vi "ORS_LinearizeFFTSingleLine - Copy.vi"(2 "Michelson fringes":dbl[](array[numeric]), 4 "Linearization method":u16=1, 5 "inverted Hilbert in":dbl[](array[numeric]), 6 "Use DLL":bool, 7 "RecalFringePhaseFit":dbl[](array[numeric]), 8 "DLL path":path=path "c:/", 12 "Window":T1=62 items=["Rectangle"=0, "Hanning"=1, "Hamming"=2, "Blackman-Harris"=3, "Exact Blackman"=4, "Blackman"=5, "Flat Top"=6, "4 Term B-Harris "=7, "7 Term B-Harris"=8, "Low Sidelobe"=9, "Blackman Nuttall"=11, "Triangle"=30, "Bartlett-Hanning"=31, "Bohman"=32, "Parzen"=33, "Welch"=34, "Kaiser"=60, "Dolph-Chebyshev"=61, "Gaussian"=62], 14 "Linearizer: Interpol. method":i32, 15 "window parameter":dbl=nan, 17 "# zeros added":i32) -> (18 "Output":dbl[](array[numeric]))   [LabVIEW 2016]
uses:
  <vilib>/Analysis/4window.llb/windowTd.ctl
  <vilib>/Analysis/2dsp.llb/Real FFT.vi
  <vilib>/Analysis/4window.llb/Symmetric Window (DBL).vi
  <vilib>/Analysis/2dsp.llb/Zero Padder (DBL).vi
  <vilib>/Analysis/NI_AALPro.lvlib
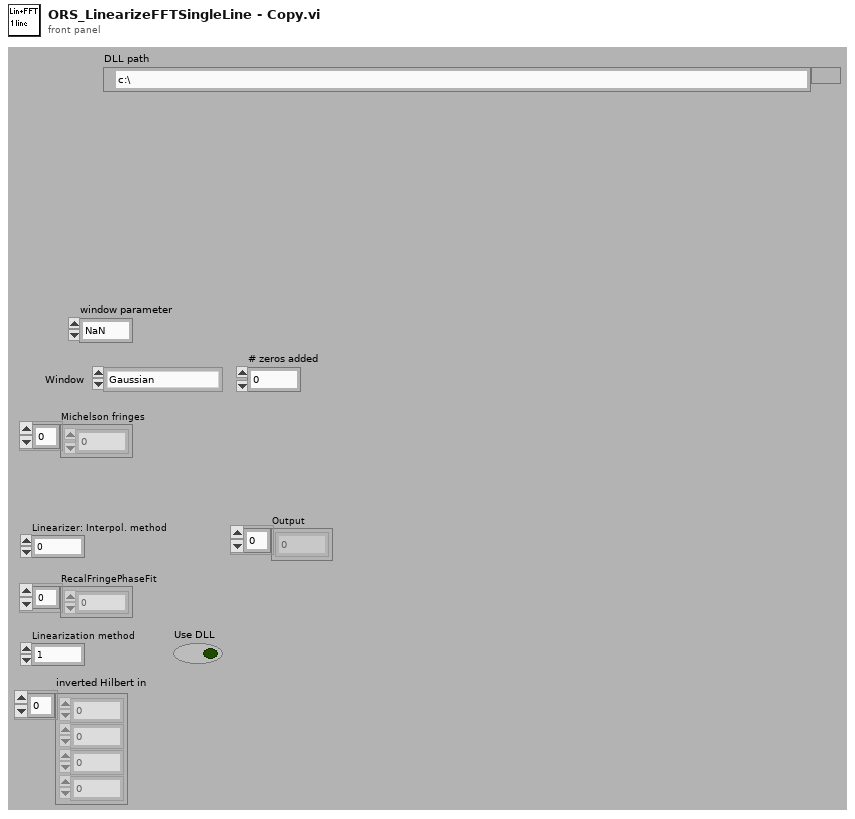
[diagram p1: front panel]
types:
  T1 = typedef "NI_AALPro.lvlib/windowTd.ctl" = u32
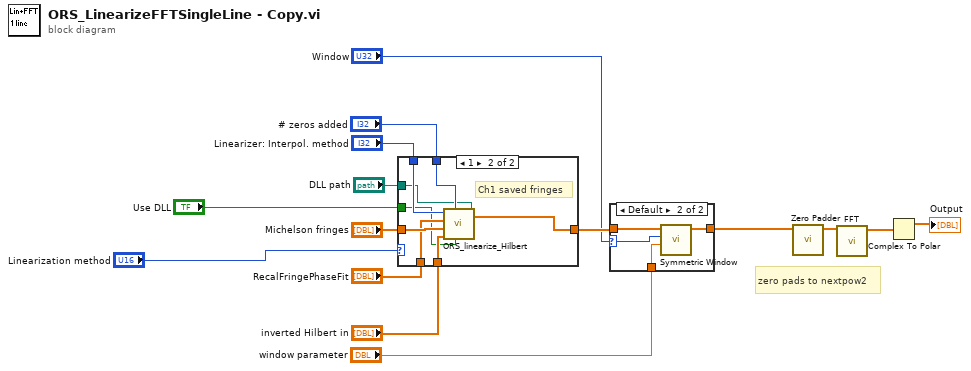
[diagram p0: block diagram]
diagram:
  # "zero pads to nextpow2"
  n1 = case shown="1" "Linearization method" {
    tunnel: [w16 w21] -> w6
    tunnel: "Linearizer: Interpol. method" -> [_ w24]
    tunnel: "Michelson fringes" -> [w16 w23]
    tunnel: "RecalFringePhaseFit" -> [_ w22]
    tunnel: "inverted Hilbert in" -> [_ w20]
    tunnel: "Use DLL" -> [_ w19]
    tunnel: "# zeros added" -> [_ w18]
    tunnel: "DLL path" -> [_ w17]
    frame 0, Default {
      # "No recalibration"
    }
    frame 1 {
      # "Ch1 saved fringes"
      n2 = call "ORS_linearize_Hilbert.vi"("DLL path"=w17, "Use DLL"=w19, "# zeros added"=w18, "inverted Hilbert in"=w20, "Ch1 Michelson"=w23, "Hilbert in"=w22, "interpolation method"=w24) -> ("Ch1 linearized"=w21:dbl[])  [unwired: 3 in, 1 out]
    }
  }
  n3 = case shown="Default" "Window" {
    selector: "Window" -> [_ w27]
    tunnel: [w25 w29] -> w2
    tunnel: w6 -> [w25 w28]
    tunnel: "window parameter" -> [_ w26]
    frame 0 {
    }
    frame Default {
      n4 = call-poly <vilib>:"Symmetric Window.vi"("window parameter"=w26, "window"=w27, "X"=w28) -> ("Windowed X"=w29:dbl[])  [unwired: 7 in, 1 out]
    }
  }
  n5 = call-poly <vilib>:"Zero Padder.vi"("Input Array"=w2) -> ("Zero Padded Array"=w11:dbl[])  [unwired: 10 in]
  n6 = call-poly <vilib>:"FFT.vi"("X"=w11) -> ("FFT {X}"=w10:cdb[])  [unwired: 9 in, 1 out]
  n7 = Complex To Polar(r * e^(i*theta)=w10) -> (r=→"Output":dbl[])  [unwired: 1 out]
